vi "Find Library Path.vi"(7 "Library Name":string="TimingDRV Engine.lvlib", 8 "error in (no error)":errorcluster, 10 "Target Name":string="My Computer", 11 "Project Sync Tools in":refnum<class "Project Sync Tools.lvclass">) -> (0 "error out":errorcluster, 1 "Found":bool, 2 "Library Path":path, 3 "Project Sync Tools out":refnum<class "Project Sync Tools.lvclass">)   [LabVIEW 2019, in "Project Sync Tools.lvclass"]
uses:
  Project Sync Tools.lvclass
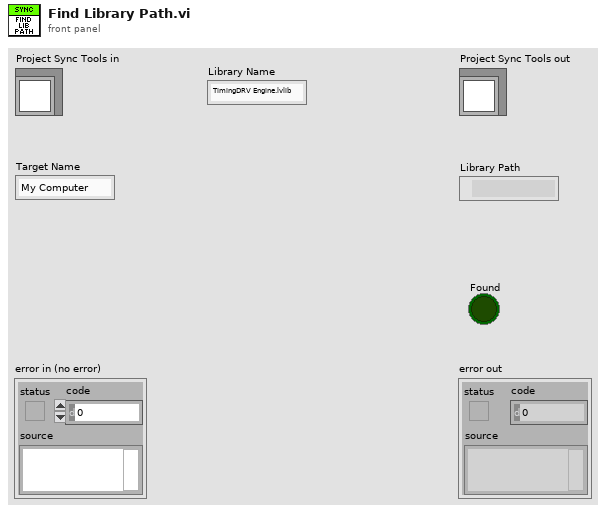
[diagram p1: front panel]
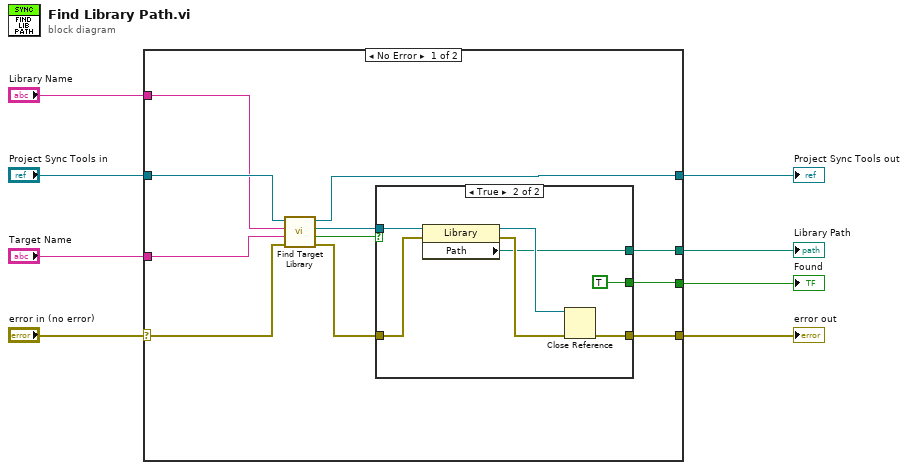
[diagram p0: block diagram]
diagram:
  n1 = case shown="No Error" "error in (no error)" {
    selector: "error in (no error)" -> [w15 w29]
    tunnel: [w14 w29] -> w7
    tunnel: [w16 w28] -> w5
    tunnel: "Project Sync Tools in" -> [w17 w28]
    tunnel: "Target Name" -> [w10 _]
    tunnel: "Library Name" -> [w9 _]
    tunnel: [w12 _] -> w4
    tunnel: [w11 _] -> w3
    frame No Error {
      n2 = call "Find Target Library.vi"("error in (no error)"=w15, "Target Name"=w10, "Library Name"=w9, "CD Build Tools in"=w17) -> ("error out"=w19:errorcluster, "Found ?"=w13:bool, "Library out"=w18:refnum<vi>, "CD Build Tools out"=w16:refnum<class "Project Sync Tools.lvclass">)  [unwired: 4 in]
      n3 = case shown="True" w13 {
        tunnel: w19 -> [w20 w25]
        tunnel: w18 -> [_ w24]
        tunnel: [w20 w23] -> w14
        tunnel: [_ w22] -> w12
        tunnel: [_ TRUE] -> w11
        frame False {
        }
        frame True {
          n4 = property class="Library"(reference=w24, error in=w25) -> (reference out=w27:refnum<vi>, error out=w26:errorcluster, "Path"=w22:path)
          n5 = Close Reference(reference=w27, error in (no error)=w26) -> (error out=w23:errorcluster)
        }
      }
    }
    frame Error {
    }
  }
  "error out" <- w7
  "Project Sync Tools out" <- w5
  "Library Path" <- w4
  "Found" <- w3
